vi "Compressor Loop.vi"(10 "CompressorDevRef":T2={"DevStatus"={"status"=FALSE, "code"=0, "source"=""}, "DigitalInputDevRef"={"DevStatus"={"status"=FALSE, "code"=0, "source"=""}, "DIO Channel"=enum."Invalid", "Digital Module"=enum."Digital Module 1"}, "RelayDevRef"={"DevStatus"={"status"=FALSE, "code"=0, "source"=""}, "Relay Channel"=enum."Invalid", "Digital Module"=enum."Digital Module 1", "Relay Direction"=enum."Both directions"}}) -> ()   [LabVIEW 2013]
uses:
  <vilib>/Rock Robotics/WPI/Compressor/WPI_CompressorDevRef.ctl
  <vilib>/Rock Robotics/WPI/DigitalInput/WPI_DigitalInputDevRef.ctl
  <vilib>/Rock Robotics/SystemInterfaces/DIO/FPGA_DIOChannel.ctl
  <vilib>/Rock Robotics/SystemInterfaces/Typedef/FPGA_TypedefDigitalModule.ctl
  <vilib>/Rock Robotics/WPI/Relay/WPI_RelayDevRef.ctl
  <vilib>/Rock Robotics/SystemInterfaces/DIO/FPGA_DIORelayChannel.ctl
  <vilib>/Rock Robotics/WPI/Relay/WPI_RelayDirection.ctl
  Compressor State.ctl
  <vilib>/Rock Robotics/WPI/Relay/WPI_RelayValue.ctl
  Common Code/Change Detect Int.vi
  Robot Global Data.vi
  <vilib>/Rock Robotics/WPI/AnalogModule/WPI_AnalogModuleGetAverageVoltage.vi
  <vilib>/Utility/error.llb/Clear Errors.vi
panel:
  out "Compressor":bool
  in  "Switch":bool
  in  "Low Volt":bool
  out "State":T1=enum."Full"
  in  "error in (no error)":errorcluster
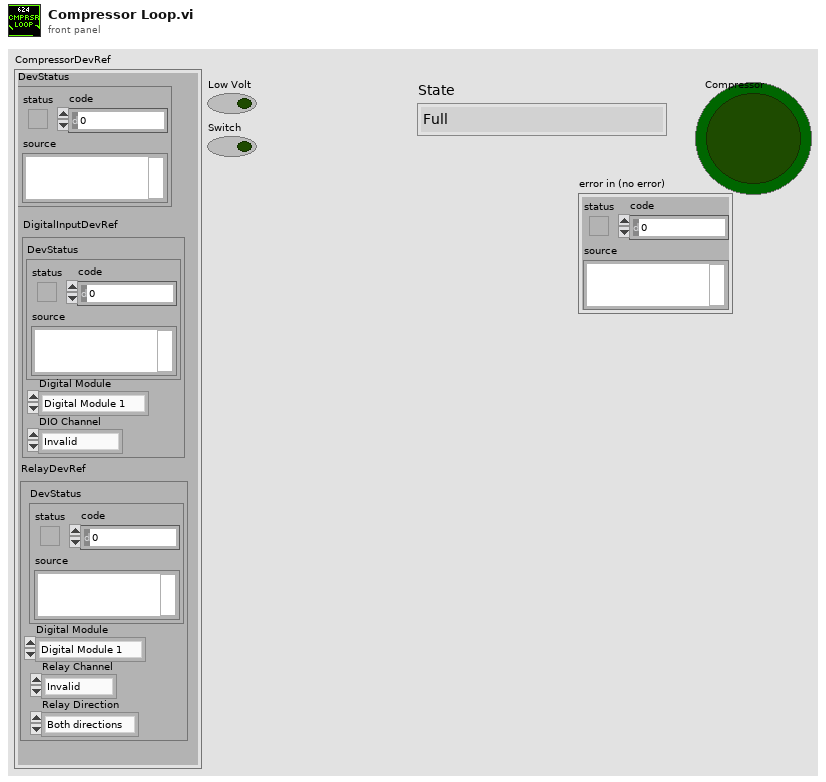
[diagram p1: front panel]
types:
  T1 = typedef "Compressor State.ctl" = enum16{"Cutoff Wait", "Running", "Full", "Low Voltage", "Voltage Wait"}
  T2 = typedef "WPI_CompressorDevRef.ctl" = cluster{"DevStatus":errorcluster, "DigitalInputDevRef":T3, "RelayDevRef":T6}
  T3 = typedef "WPI_DigitalInputDevRef.ctl" = cluster{"DevStatus":errorcluster, "DIO Channel":T4, "Digital Module":T5}
  T4 = typedef "FPGA_DIOChannel.ctl" = enum8{"DIO 1", "DIO 2", "DIO 3", "DIO 4", "DIO 5", "DIO 6", "DIO 7", "DIO 8", "DIO 9", "DIO 10", "DIO 11", "DIO 12", "DIO 13", "DIO 14", "Invalid"}
  T5 = typedef "FPGA_TypedefDigitalModule.ctl" = enum16{"Digital Module 1", "Digital Module 2"}
  T6 = typedef "WPI_RelayDevRef.ctl" = cluster{"DevStatus":errorcluster, "Relay Channel":T7, "Digital Module":T5, "Relay Direction":T8}
  T7 = typedef "FPGA_DIORelayChannel.ctl" = enum8{"Relay 1", "Relay 2", "Relay 3", "Relay 4", "Relay 5", "Relay 6", "Relay 7", "Relay 8", "Invalid"}
  T8 = typedef "WPI_RelayDirection.ctl" = enum16{"Both directions", "Forward only", "Reverse only"}
  T9 = typedef "WPI_RelayValue.ctl" = enum16{"Off", "On", "Forward", "Reverse"}
  T10 = typedef "Dashboard UDP Packet.ctl" = cluster{"Camera":T11, "Gyro":T12, "Encoder":T14, "Auto Shift":T15, "Auton":T16, "Drive/Ramp X":dbl, "Drive/Ramp Y":dbl, "Drive/Battery Cutoff":dbl, "Pressure/Compressor Min Voltage":dbl, "Pressure/Compressor Delay":dbl, "Controller/Strafe Correction":bool, "Shooter":T17, "Rollers":T18, "Abort":bool, "Finish":bool, "Shooter Halo Time":dbl, "IR Halo Sustain Time":dbl, "Disable Compressor":bool}
  T11 = typedef "Camera Controls.ctl" = cluster{"Camera/View Angle X":dbl, "Camera/Goal Track Timeout":dbl, "Camera/View Angle Y":dbl, "Camera/Goal Exposure":dbl, "Camera/Vision Receive Timeout":dbl, "Camera/Offset 1":dbl, "Camera/Offset 2":dbl}
  T12 = typedef "Gyro Controls.ctl" = cluster{"Gyro/Angle Tolerance":dbl, "Gyro/Steer Closeness Threshold":dbl, "Steer PID":T13, "Steer Close PID":T13}
  T13 = typedef "PID Params.ctl" = cluster{"max":dbl, "min":dbl, "P":dbl, "I":dbl, "D":dbl}
  T14 = typedef "Encoder Controls.ctl" = cluster{"Encoders/Reset":bool, "Encoders/Omni Constant":dbl, "Encoders/Omni Tick Constant":dbl, "Encoders/Left Constant":dbl, "Encoders/Right Constant":dbl, "Encoders/Right Tick Constant":dbl}
  T15 = typedef "Auto Shift Controls.ctl" = cluster{"AutoShift/Upshift Throttle Accel":dbl, "AutoShift/Speed Threshold":dbl, "AutoShift/Upshift Throttle":dbl, "AutoShift/Upshift Accel":dbl, "AutoShift/Downshift Accel":dbl, "AutoShift/Downshift Throttle":dbl, "AutoShift/Delay":dbl, "AutoShift/Enabled":bool}
  T16 = typedef "Auton Controls.ctl" = cluster{"Auton/Left Shoot X-Coord":dbl, "Auton/Right Shoot X-Coord":dbl, "DistDrive/Distance Stop Threshold":dbl, "DistDrive/Max Stop Speed":dbl, "Auton/Back Piston Time":dbl, "Auton/Manual Hot":bool, "Auton/Manual Hot Right":bool, "Default X PID":T13, "Default Y PID":T13}
  T17 = typedef "Shooter Controls.ctl" = cluster{"Shooter/Reset Time":dbl, "Shooter/Release Delay":dbl, "Shooter/Pressure Steady Time":dbl, "Shooter/Misfire Delay":dbl, "Shooter/Ball Settle Time":dbl, "Shooter/Line IR Delay":dbl, "Pressure/Upper PSI Time":dbl, "Pressure/Lower PSI Time":dbl, "Shooter/Punch Delay":dbl, "Shooter/Target Pressure":dbl, "Pressure/Line B":dbl, "Pressure/Line M":dbl, "Pressure/Shooter M":dbl, "Pressure/Shooter B":dbl}
  T18 = typedef "Roller Controls.ctl" = cluster{"Roller/Load IRs Verify Time":dbl, "Roller/Center IR Latch Time":dbl, "Roller/Speed Front":dbl, "Roller/Speed Back":dbl, "Roller/Entry Timeout":dbl, "Roller/To Center Timeout":dbl, "Roller/Sustain Time":dbl, "Roller/Verify Center Time":dbl}
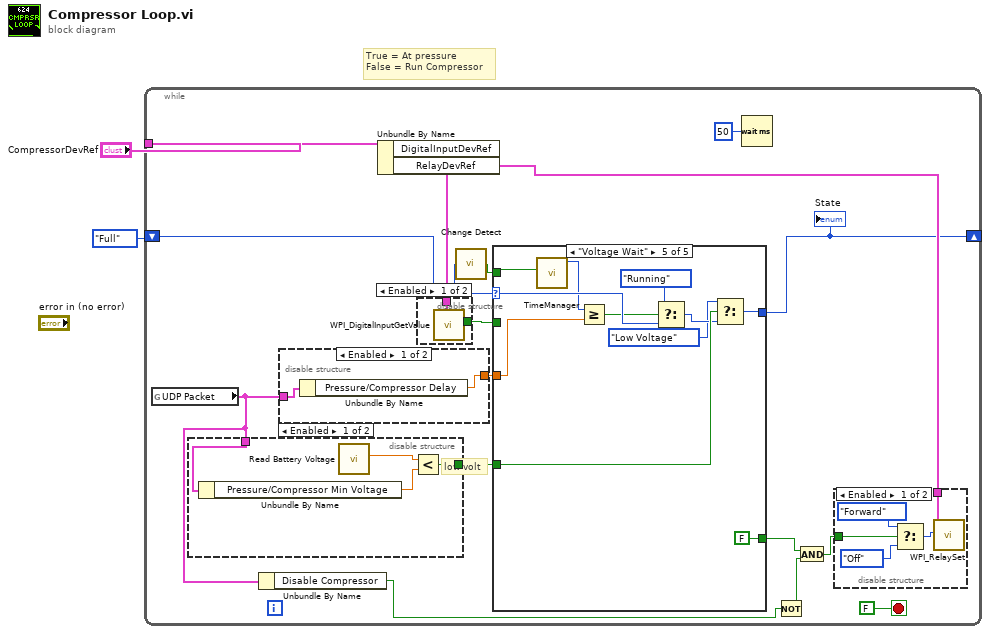
[diagram p0: block diagram]
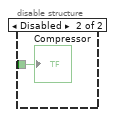
[diagram p2: hidden frame]
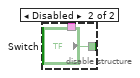
[diagram p3: hidden frame]
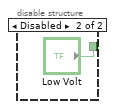
[diagram p4: hidden frame]
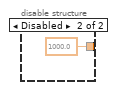
[diagram p5: hidden frame]
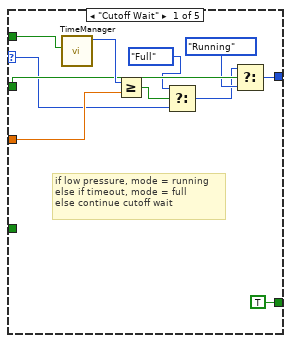
[diagram p6: hidden frame]
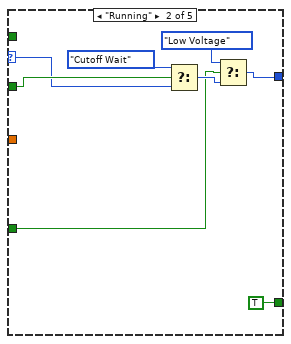
[diagram p7: hidden frame]
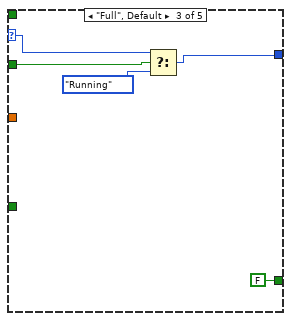
[diagram p8: hidden frame]
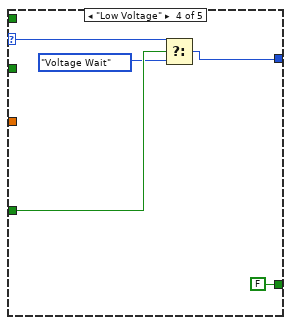
[diagram p9: hidden frame]
diagram:
  # "True = At pressure\nFalse = Run Compressor"
  n1 = while {
    tunnel: "CompressorDevRef" -> [w18]
    shift-right: [w14] -> _
    shift-left: Compressor_State."Full" ("State") -> [w13]
    stop <- FALSE stop-if-true
    n2 = global read "Robot Global Data.vi" "UDP Packet"() -> (w7:T10)
    n3 = disable-structure shown="Enabled" {
      disable-tunnel: [w30 "Low Volt"] -> w10
      disable-tunnel: w7 -> [w28 _]
      frame Enabled {
        # "low volt"
        n4 = Unbundle By Name(w28) -> ("Pressure/Compressor Min Voltage"=w29:dbl)
        n5 = call "Read Battery Voltage.vi"() -> ("Voltage"=w31:dbl)  [unwired: 11 in]
        n6 = Less?(x=w31, y=w29) -> (x < y?=w30:bool)
      }
      frame Disabled {
      }
    }
    n7 = Unbundle By Name(w7) -> ("Disable Compressor"=w6:bool)
    n8 = disable-structure shown="Enabled" {
      disable-tunnel: [w33 1000.0 ("Numeric")] -> w11
      disable-tunnel: w7 -> [w34 _]
      frame Enabled {
        n9 = Unbundle By Name(w34) -> ("Pressure/Compressor Delay"=w33:dbl)
      }
      frame Disabled {
      }
    }
    n10 = Unbundle By Name(w18) -> ("DigitalInputDevRef"=w17:T3, "RelayDevRef"=w16:T6)
    n11 = disable-structure shown="Enabled" {
      disable-tunnel: w17 -> [w26 _]
      disable-tunnel: [w25 "Switch"] -> w15
      frame Enabled {
        n12 = call <vilib>:"WPI_DigitalInputGetValue.vi"("DigitalInputDevRef"=w26) -> ("Value"=w25:bool)  [unwired: 1 in, 9 out]
      }
      frame Disabled {
      }
    }
    n13 = call-poly "Change Detect.vi"("In"=w13) -> ("Changed?"=w12:bool)
    n14 = case shown="\"Voltage Wait\"" w13 {
      selector: w13 -> [w36 w52 w57 w62 w75]
      tunnel: [TRUE TRUE FALSE FALSE FALSE] -> w4
      tunnel: w15 -> [w43 w53 w58 _ _]
      tunnel: [w41 w48 w56 w61 w69] -> w14
      tunnel: w12 -> [w46 _ _ _ w74]
      tunnel: w11 -> [w44 _ _ _ w72]
      tunnel: w10 -> [_ w49 _ w63 w68]
      frame "Cutoff Wait" {
        # "if low pressure, mode = running\nelse if timeout, mode = full\nelse continue cutoff wait"
        n15 = call "TimeManager.vi"("Reset?"=w46) -> ("Time Since Reset"=w45:u32)  [unwired: 9 in, 1 out]
        n16 = Greater Or Equal?(x=w45, y=w44) -> (x >= y?=w38:bool)
        n17 = Select(t=Compressor_State."Full" ("State"), s=w38, f=w36) -> (s? t:f=w39:T1)
        n18 = Select(t=w39, s=w43, f=Compressor_State."Running") -> (s? t:f=w41:T1)
      }
      frame "Running" {
        n19 = Select(t=Compressor_State."Cutoff Wait" ("State"), s=w53, f=w52) -> (s? t:f=w50:T1)
        n20 = Select(t=Compressor_State."Low Voltage", s=w49, f=w50) -> (s? t:f=w48:T1)
      }
      frame "Full", Default {
        n21 = Select(t=w57, s=w58, f=Compressor_State."Running") -> (s? t:f=w56:T1)
      }
      frame "Low Voltage" {
        n22 = Select(t=w62, s=w63, f=Compressor_State."Voltage Wait") -> (s? t:f=w61:T1)
      }
      frame "Voltage Wait" {
        n23 = call "TimeManager.vi"("Reset?"=w74) -> ("Time Since Reset"=w73:u32)  [unwired: 9 in, 1 out]
        n24 = Greater Or Equal?(x=w73, y=w72) -> (x >= y?=w71:bool)
        n25 = Select(t=Compressor_State."Running", s=w71, f=w75) -> (s? t:f=w67:T1)
        n26 = Select(t=Compressor_State."Low Voltage", s=w68, f=w67) -> (s? t:f=w69:T1)
      }
    }
    "State" <- w14
    n27 = Wait (ms)(milliseconds to wait=u32 50) -> ()  [unwired: 1 out]
    n28 = Not(x=w6) -> (.not. x?=w5:bool)
    n29 = And(x=w4, y=w5) -> (x .and. y?=w3:bool)
    n30 = disable-structure shown="Enabled" {
      disable-tunnel: w16 -> [w23 _]
      disable-tunnel: w3 -> [w19 w24]
      frame Enabled {
        n31 = Select(t=WPI_RelayValue."Forward" ("RelayValue"), s=w19, f=WPI_RelayValue."Off" ("RelayValue")) -> (s? t:f=w22:T9)
        n32 = call <vilib>:"WPI_RelaySet.vi"("RelayValue"=w22, "RelayDevRef"=w23) -> ()  [unwired: 1 in, 9 out]
      }
      frame Disabled {
        "Compressor" <- w24
      }
    }
  }
